vi "SRV_Read JPG.vi"(8 "error in":errorcluster, 9 "timeout ms (25000)":i32=25000, 10 "Header Info In":string, 11 "connection ID in":refnum<k5>) -> (0 "error out":errorcluster, 1 "data out":string, 3 "connection ID":refnum<k5>)   [LabVIEW 2014]
panel:
  out "size":u32
  out "rest of header (hex display)":string
  out "first char after ##IMJ":string
  out "before ##IMJ":string
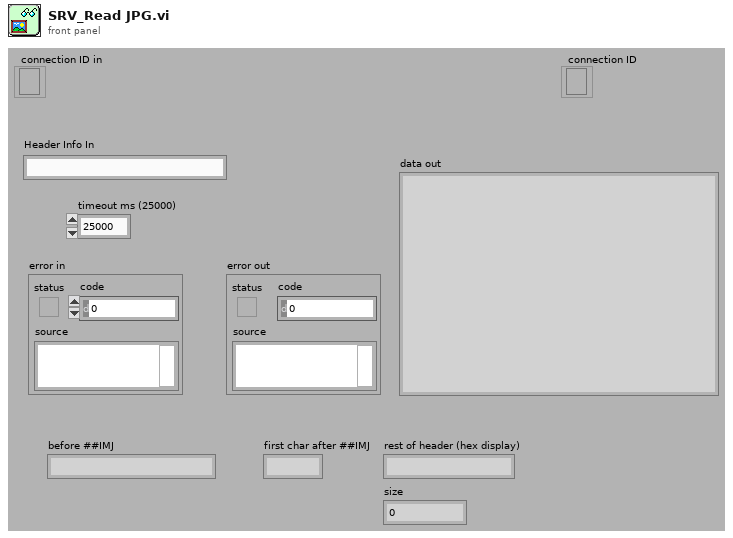
[diagram p1: front panel]
types:
  T1 = typedef "SRV_PM_Packet Mode Style.ctl" = enum16{"Old", "New PM"}
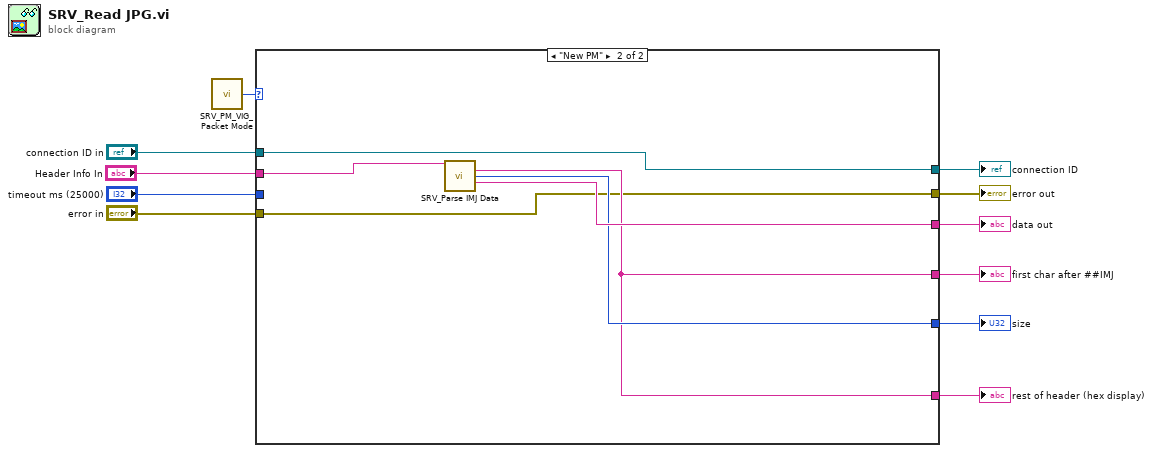
[diagram p0: block diagram]
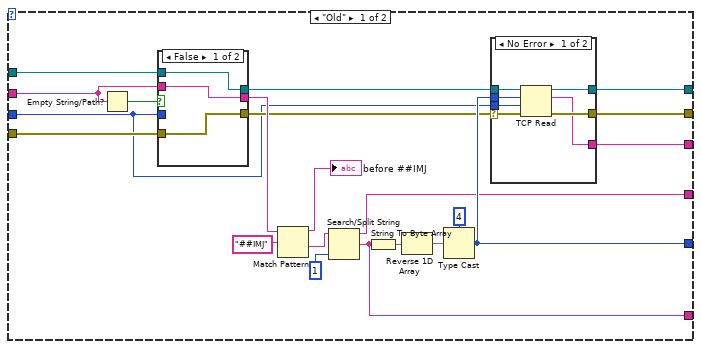
[diagram p2: hidden frame]
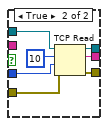
[diagram p3: hidden frame]
diagram:
  n1 = call "SRV_PM_VIG_Packet Mode.vi"() -> ("Packet Mode Style"=w2:T1)  [unwired: 15 in]
  n2 = case shown="\"New PM\"" w2 {
    tunnel: "error in" -> [w32 w52]
    tunnel: "connection ID in" -> [w31 w56]
    tunnel: [w24 w54] -> w9
    tunnel: [w23 w53] -> w8
    tunnel: [w22 w56] -> w7
    tunnel: [w21 w52] -> w6
    tunnel: [w19 w55] -> w5
    tunnel: "Header Info In" -> [w14 w57]
    tunnel: "timeout ms (25000)" -> [w13 _]
    tunnel: [w12 w53] -> w1
    frame "Old" {
      n3 = Empty String/Path?(string/path=w14) -> (empty?=w15:bool)
      n4 = case shown="False" w15 {
        tunnel: w32 -> [w33 w42]
        tunnel: w31 -> [w35 w41]
        tunnel: [w34 w40] -> w26
        tunnel: [w35 w39] -> w25
        tunnel: [w33 w38] -> w20
        tunnel: w13 -> [_ w37]
        tunnel: w14 -> [w34 _]
        frame False {
        }
        frame True {
          n5 = TCP Read(connection ID=w41, bytes to read=10, error in (no error)=w42, 9:w37) -> (connection ID out=w39:refnum<k5>, data out=w40:string, error out=w38:errorcluster)  [unwired: 1 in]
        }
      }
      n6 = Match Pattern(string=w26, regular expression="##IMJ") -> (before substring=→"before ##IMJ":string, after substring=w17:string)  [unwired: 1 in, 2 out]
      n7 = Search/Split String(string=w17, offset (0)=1) -> (substring before match=w12:string, match + rest of string=w23:string)  [unwired: 1 in, 1 out]
      n8 = String To Byte Array(string=w23) -> (unsigned byte array=w29:u8[])
      n9 = Reverse 1D Array(array=w29) -> (reversed array=w27:u8[])
      n10 = Type Cast(type=u32 4 ("offset (0)"), x=w27) -> (*(type *) &x=w24:u32)
      n11 = case shown="No Error" w20 {
        selector: w20 -> [w43 w50]
        tunnel: w25 -> [w49 w51]
        tunnel: w24 -> [w48 _]
        tunnel: [w47 w51] -> w22
        tunnel: [w46 w50] -> w21
        tunnel: [w45 _] -> w19
        tunnel: w13 -> [w44 _]
        frame No Error {
          n12 = TCP Read(connection ID=w49, bytes to read=w48, error in (no error)=w43, 9:w44) -> (connection ID out=w47:refnum<k5>, data out=w45:string, error out=w46:errorcluster)  [unwired: 1 in]
        }
        frame Error {
        }
      }
    }
    frame "New PM" {
      n13 = call "SRV_Parse IMJ Data.vi"("##IMJ Data"=w57) -> ("frame size in pixels"=w53:string, "Frame Size in Bytes"=w54:u32, "Rest of frame data"=w55:string)  [unwired: 12 in]
    }
  }
  "data out" <- w5
  "rest of header (hex display)" <- w8
  "error out" <- w6
  "connection ID" <- w7
  "size" <- w9
  "first char after ##IMJ" <- w1
